vi "PRIOR_IFilterClose.vi"(8 "error in (no error)":errorcluster, 11 "PRIORLib In":T1) -> (0 "error out":errorcluster)   [LabVIEW 2010]
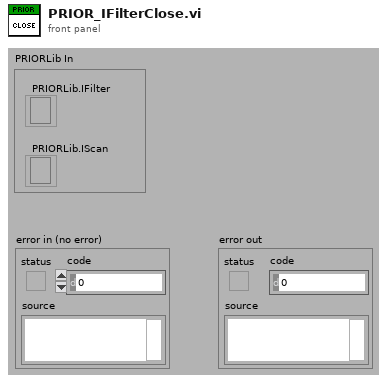
[diagram p1: front panel]
types:
  T1 = cluster{"PRIORLib.IFilter":refnum<k7>, "PRIORLib.IScan":refnum<k7>}
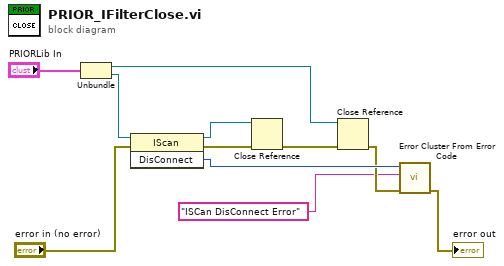
[diagram p0: block diagram]
diagram:
  n1 = Unbundle("PRIORLib In") -> ("PRIORLib.IFilter"=w1:refnum<k7>, "PRIORLib.IScan"=w10:refnum<k7>)
  n2 = invoke class="IScan" method="DisConnect"(reference=w10, error in="error in (no error)") -> (reference out=w6:refnum<k7>, error out=w7:errorcluster, "DisConnect"=w5:i32)  [unwired: 1 in]
  n3 = Close Reference(reference=w6, error in (no error)=w7) -> (error out=w8:errorcluster)
  n4 = Close Reference(reference=w1, error in (no error)=w8) -> (error out=w4:errorcluster)
  n5 = call <vilib>:"Error Cluster From Error Code.vi"("error in (no error)"=w4, "error message (\"\")"="ISCan DisConnect Error" ("error message (\"\")"), "error code (0)"=w5) -> ("error out"=→"error out":errorcluster)  [unwired: 6 in]
